vi "Read UI elements.vi"(11 "Controller in":refnum<class "Controller.lvclass">) -> (2 "UI elements":T1, 3 "Controller out":refnum<class "Controller.lvclass">)   [LabVIEW 2011, in "Controller.lvclass"]
uses:
  Controller.lvclass
  Controls/UI Elements.ctl
  Controller.lvclass/Controller.ctl
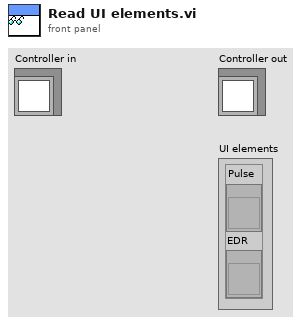
[diagram p1: front panel]
types:
  T1 = typedef "Controller.lvclass/UI Elements.ctl" = cluster{"Pulse":refnum<vi>, "EDR":refnum<vi>}
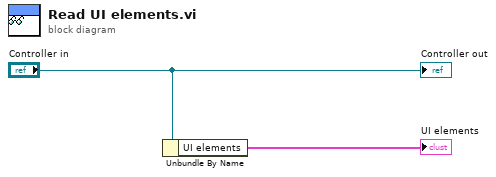
[diagram p0: block diagram]
diagram:
  n1 = Unbundle By Name("Controller in") -> ("UI elements"=→"UI elements":T1)
  "Controller out" <- "Controller in"
